vi "rs.vi"(2 "error out":errorcluster, 3 "字符串":string, 4 "delay before read (ms)":u32=500 caption="读取前延时(ms)", 5 "VISA resource name out":refnum<visa-resource-name>) -> (0 "read string":string caption="读取字符串")   [LabVIEW 2009]
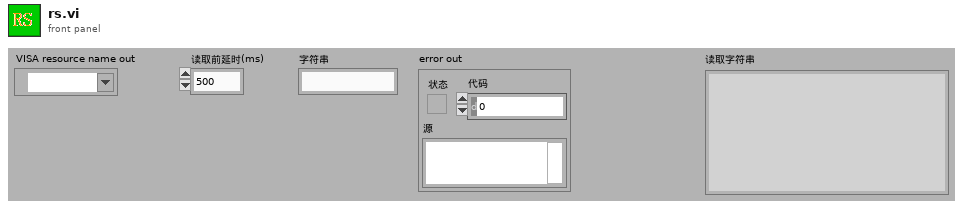
[diagram p1: front panel]
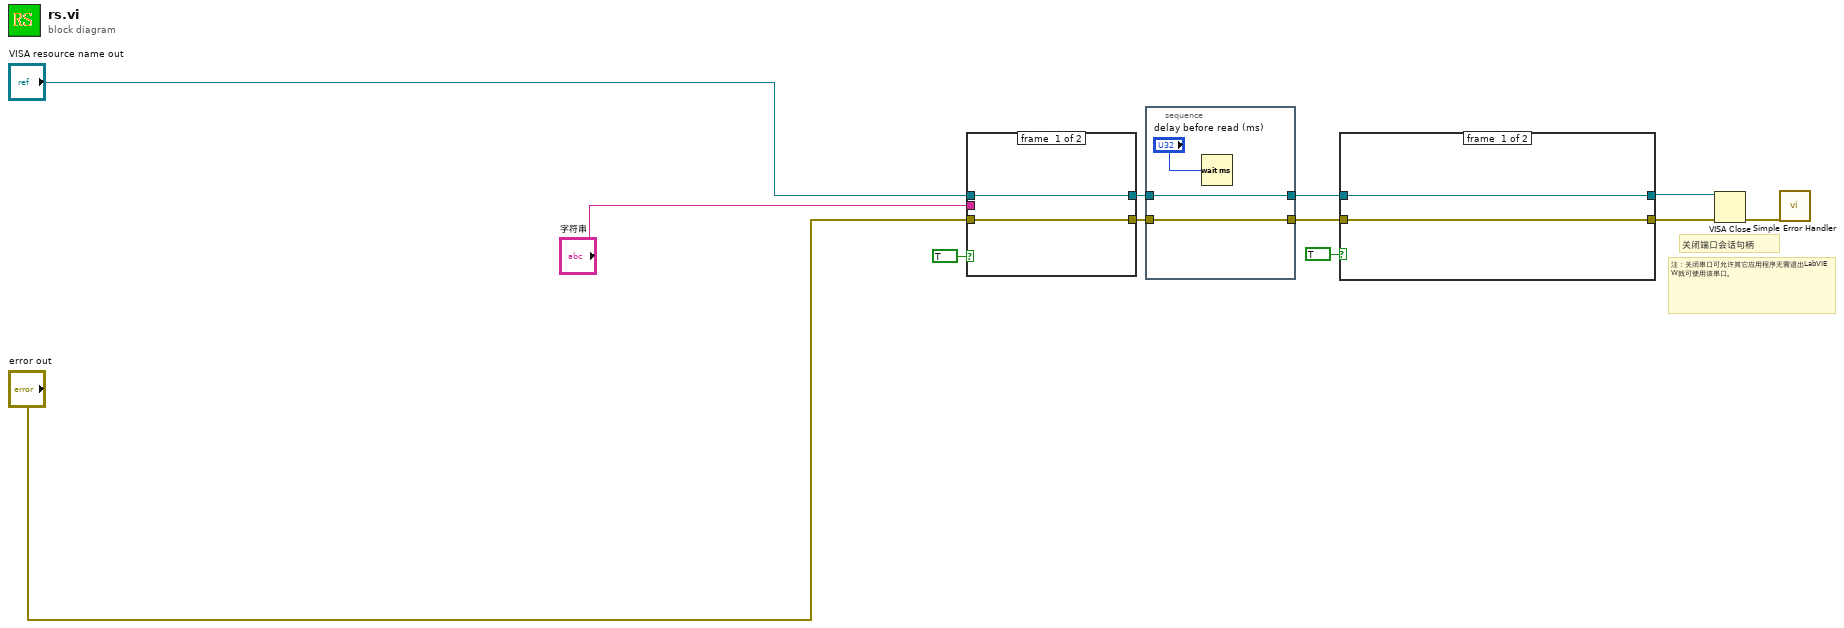
[diagram p0: block diagram]
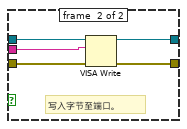
[diagram p2: hidden frame]
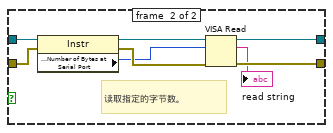
[diagram p3: hidden frame]
diagram:
  # "注：关闭串口可允许其它应用程序无需退出LabVIEW就可使用该串口。"
  # "关闭端口会话句柄"
  n1 = case shown="真" TRUE {
    tunnel: [w14 w19] -> w7
    tunnel: "VISA resource name out" -> [w13 w18]
    tunnel: "error out" -> [w14 w17]
    tunnel: [w13 w16] -> w9
    tunnel: "字符串" -> [_ w15]
    frame #0 {
    }
    frame #1 {
      # "写入字节至端口。"
      n2 = VISA Write(VISA resource name=w18, write buffer=w15, error in (no error)=w17) -> (VISA resource name out=w16:refnum<visa-resource-name>, error out=w19:errorcluster)  [unwired: 1 out]
    }
  }
  n3 = stacked-sequence {
    tunnel: w7 -> [w22]
    tunnel: [w22] -> w8
    tunnel: w9 -> [w21]
    tunnel: [w21] -> w10
    frame #0 {
      n4 = Wait (ms)(milliseconds to wait="delay before read (ms)") -> ()  [unwired: 1 out]
    }
  }
  n5 = case shown="真" TRUE {
    tunnel: w8 -> [w24 w28]
    tunnel: [w24 w32] -> w4
    tunnel: [w23 w31] -> w5
    tunnel: w10 -> [w23 w30]
    frame #0 {
    }
    frame #1 {
      # "读取指定的字节数。"
      n6 = property class="Instr"(reference=w30, error in=w28) -> (reference out=w29:refnum<visa-resource-name>, error out=w27:errorcluster, "Serial Settings:Number of Bytes at Serial Port"=w25:u32)
      n7 = VISA Read(VISA resource name=w29, byte count=w25, error in (no error)=w27) -> (VISA resource name out=w31:refnum<visa-resource-name>, read buffer=→"read string":string, error out=w32:errorcluster)  [unwired: 1 out]
    }
  }
  n8 = VISA Close(VISA resource name=w5, error in (no error)=w4) -> (error out=w6:errorcluster)
  n9 = call <vilib>:"Simple Error Handler.vi"("error in (no error)"=w6) -> ()  [unwired: 1 in, 8 out]
